vi "Sound Tester.vi"() -> ()   [LabVIEW 2019]
uses:
  Sound.lvclass
panel:
  in  "stop":bool
  in  "Sound Parameters":T1={"Device ID"=0, "Volume"=50.0, "frequency"=10.0, "duration (s)"=0.0} {"frequency" format="%0.2p"; "Volume" scale=0.0..100.0}
  in  "error in (no error)":errorcluster
  out "error out":errorcluster
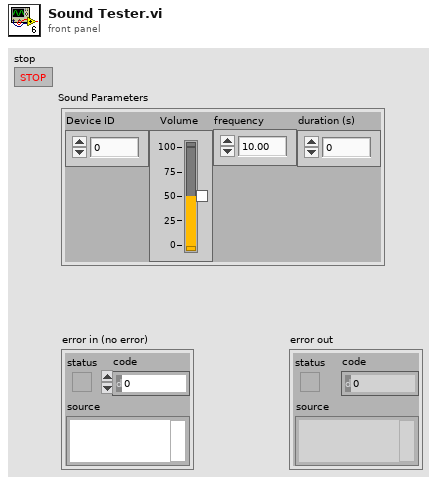
[diagram p1: front panel]
types:
  T1 = cluster{"Device ID":u32, "Volume":dbl, "frequency":dbl, "duration (s)":dbl}
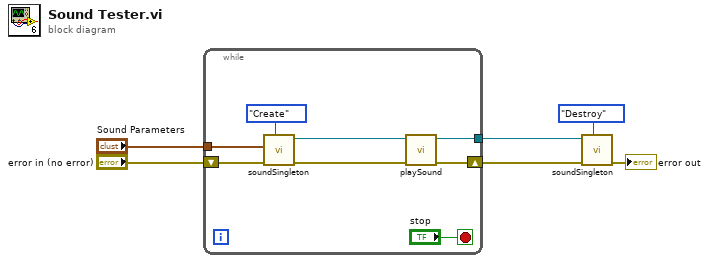
[diagram p0: block diagram]
diagram:
  n1 = while {
    tunnel: [w11] -> w4
    tunnel: "Sound Parameters" -> [w9]
    shift-right: [w12] -> w6
    shift-left: "error in (no error)" -> [w10]
    stop <- "stop" stop-if-true
    n2 = call "soundSingleton.vi"("Option"=enum16{"Create", "Destroy"}."Create", "error in (no error)"=w10, "Sound Parameters"=w9) -> ("error out"=w13:errorcluster, "Sound out"=w14:refnum<class "Sound.lvclass">)  [unwired: 7 in]
    n3 = call "playSound.vi"("error in (no error)"=w13, "Sound in"=w14) -> ("error out"=w12:errorcluster, "Sound out"=w11:refnum<class "Sound.lvclass">)  [unwired: 8 in]
  }
  n4 = call "soundSingleton.vi"("Option"=enum16{"Create", "Destroy"}."Destroy", "error in (no error)"=w6, "Sound in"=w4) -> ("error out"=→"error out":errorcluster)  [unwired: 7 in, 1 out]
